vi "FL Fuzzy Controller (MIMO).vi"(8 "error in (no error)":errorcluster, 10 "input values":dbl[](array[numeric]), 11 "fuzzy system in":T1 {"user MF interpolating polynomials"."coa_x(y) coeff" format="%.4g"; "user MF interpolating polynomials"."Area(y) coeff" format="%.4g"; "user MF interpolating polynomials"."X(y) coeff" format="%.4g"; "user MF interpolating polynomials"."Y(x) coeff" format="%.4g"; "user MF interpolating polynomials"."Y" format="%.4g"; "user MF interpolating polynomials"."X" format="%.4g"; "defuzzification method" items=["Center of Area", "Modified Center of Area", "Center of Sums", "Center of Maximum", "Mean of Maximum"]; "rules"."consequents"."Var Index" min=0; "rules"."consequents"."Cond" items=["=", "!="]; "rules"."consequents"."MF Index" min=0; "rules"."antecedents"."Var Index" min=0; "rules"."antecedents"."Cond" items=["=", "!="]; "rules"."antecedents"."MF Index" min=0; "rules"."consequent implication" items=["Minimum", "Product"]; "rules"."antecedent connective" items=["AND (Minimum)", "AND (Product)", "OR (Maximum)", "OR (Probabilistic)"]; "output variables"."MFs"."shape" items=["Triangle", "Trapezoid", "Singleton", "Sigmoid", "Gaussian", "User-Defined"]; "input variables"."MFs"."shape" items=["Triangle", "Trapezoid", "Singleton", "Sigmoid", "Gaussian", "User-Defined"]}) -> (0 "error out":errorcluster, 1 "rule weights":dbl[](array[numeric]), 2 "output values":dbl[](array[numeric]), 3 "fuzzy system out":T1 {"user MF interpolating polynomials"."coa_x(y) coeff" format="%.4g"; "user MF interpolating polynomials"."Area(y) coeff" format="%.4g"; "user MF interpolating polynomials"."X(y) coeff" format="%.4g"; "user MF interpolating polynomials"."Y(x) coeff" format="%.4g"; "user MF interpolating polynomials"."Y" format="%.4g"; "user MF interpolating polynomials"."X" format="%.4g"; "defuzzification method" items=["Center of Area", "Modified Center of Area", "Center of Sums", "Center of Maximum", "Mean of Maximum"]; "rules"."consequents"."Var Index" min=0; "rules"."consequents"."Cond" items=["=", "!="]; "rules"."consequents"."MF Index" min=0; "rules"."antecedents"."Var Index" min=0; "rules"."antecedents"."Cond" items=["=", "!="]; "rules"."antecedents"."MF Index" min=0; "rules"."consequent implication" items=["Minimum", "Product"]; "rules"."antecedent connective" items=["AND (Minimum)", "AND (Product)", "OR (Maximum)", "OR (Probabilistic)"]; "output variables"."MFs"."shape" items=["Triangle", "Trapezoid", "Singleton", "Sigmoid", "Gaussian", "User-Defined"]; "input variables"."MFs"."shape" items=["Triangle", "Trapezoid", "Singleton", "Sigmoid", "Gaussian", "User-Defined"]}, 5 "rule-invoked values?":bool[](array[boolean]))   [LabVIEW 2017, in "NI_Fuzzy_Logic_API.lvlib"]
doc: "Implements a fuzzy logic controller for the fuzzy system you specify."
uses:
  <vilib>/addons/Fuzzy Logic/NI_Fuzzy_Logic_API.lvlib
  <vilib>/addons/Fuzzy Logic/TypeDefs/FL System.ctl
  <vilib>/addons/Fuzzy Logic/TypeDefs/FL Variable.ctl
  <vilib>/addons/Fuzzy Logic/TypeDefs/FL Membership Function.ctl
  <vilib>/addons/Fuzzy Logic/TypeDefs/FL Membership Function Shape.ctl
  <vilib>/addons/Fuzzy Logic/TypeDefs/FL Rule.ctl
  <vilib>/addons/Fuzzy Logic/TypeDefs/FL Antecedent.ctl
  <vilib>/addons/Fuzzy Logic/TypeDefs/FL Modifier.ctl
  <vilib>/addons/Fuzzy Logic/TypeDefs/FL Antecedent Connective.ctl
  <vilib>/addons/Fuzzy Logic/TypeDefs/FL Consequent.ctl
  <vilib>/addons/Fuzzy Logic/TypeDefs/FL Consequent Implication.ctl
  <vilib>/addons/Fuzzy Logic/TypeDefs/FL Defuzzification.ctl
  <vilib>/addons/Fuzzy Logic/TypeDefs/FL Interpolating polynomials.ctl
panel:
  # "IF"
  # "THEN"
  # "IF"
  # "THEN"
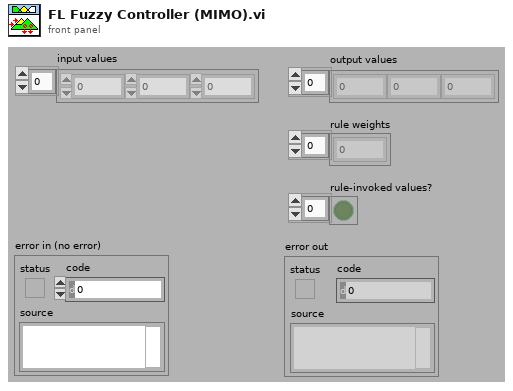
[diagram p1: front panel]
types:
  T1 = typedef "NI_Fuzzy_Logic_API.lvlib/FL System.ctl" = cluster{"input variables":T2[], "output variables":T2[], "rules":T5[], "defuzzification method":T11, "description":string, "user MF interpolating polynomials":T12[]}
  T2 = typedef "NI_Fuzzy_Logic_API.lvlib/FL Variable.ctl" = cluster{"name":string, "range":dbl[], "MFs":T3[]}
  T3 = typedef "NI_Fuzzy_Logic_API.lvlib/FL Membership Function.ctl" = cluster{"name":string, "shape":T4, "points":dbl[], "color":u32, "user-defined shape index":i32}
  T4 = typedef "NI_Fuzzy_Logic_API.lvlib/FL Membership Function Shape.ctl" = u16
  T5 = typedef "NI_Fuzzy_Logic_API.lvlib/FL Rule.ctl" = cluster{"antecedents":T6[], "antecedent connective":T8, "consequents":T9[], "consequent implication":T10, "degree of support":dbl}
  T6 = typedef "NI_Fuzzy_Logic_API.lvlib/FL Antecedent.ctl" = cluster{"Var Index":i32, "MF Index":i32, "Cond":T7}
  T7 = typedef "NI_Fuzzy_Logic_API.lvlib/FL Modifier.ctl" = u16
  T8 = typedef "NI_Fuzzy_Logic_API.lvlib/FL Antecedent Connective.ctl" = u16
  T9 = typedef "NI_Fuzzy_Logic_API.lvlib/FL Consequent.ctl" = cluster{"Var Index":i32, "MF Index":i32, "Cond":T7}
  T10 = typedef "NI_Fuzzy_Logic_API.lvlib/FL Consequent Implication.ctl" = u16
  T11 = typedef "NI_Fuzzy_Logic_API.lvlib/FL Defuzzification.ctl" = u16
  T12 = typedef "NI_Fuzzy_Logic_API.lvlib/FL Interpolating polynomials.ctl" = cluster{"X":dbl[], "Y":dbl[], "Y(x) coeff":dbl[][], "X(y) coeff":dbl[][], "Area(y) coeff":dbl[][], "coa_x(y) coeff":dbl[][]}
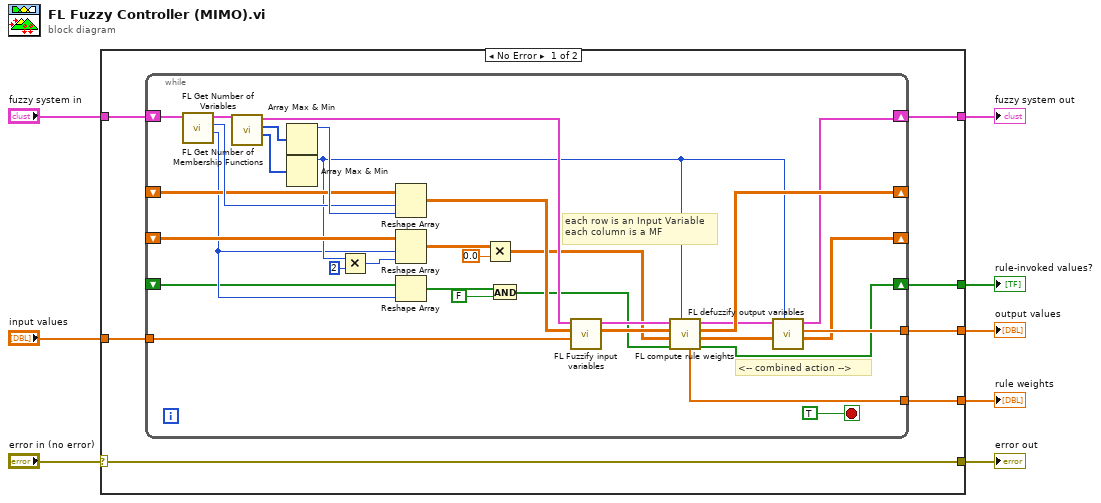
[diagram p0: block diagram]
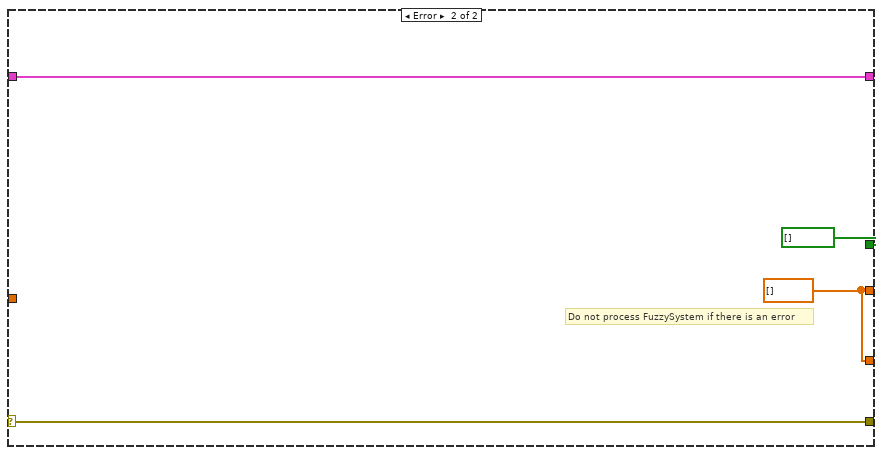
[diagram p2: hidden frame]
diagram:
  n1 = case shown="No Error" "error in (no error)" {
    selector: "error in (no error)" -> [w14 w51]
    tunnel: "fuzzy system in" -> [w12 w52]
    tunnel: [w15 w50] -> w7
    tunnel: [w14 w51] -> w6
    tunnel: [w10 w52] -> w4
    tunnel: "input values" -> [w13 _]
    tunnel: [w11 w50] -> w2
    tunnel: [w9 bool[] [] ("Array 2")] -> w1
    frame No Error {
      n2 = while {
        tunnel: [w44] -> w15
        tunnel: w13 -> [w47]
        shift-right: [w34] -> _
        shift-left: _ -> [w37]
        tunnel: [w43] -> w11
        shift-right: [w32] -> _
        shift-left: _ -> [w35]
        shift-right: [w28] -> w10
        shift-left: w12 -> [w38]
        shift-right: [w19] -> w9
        shift-left: _ -> [w20]
        stop <- TRUE stop-if-true
        # "<-- combined action -->"
        # "each row is an Input Variable\neach column is a MF"
        n3 = call <vilib>:"FL Get Number of Variables.vi"("fuzzy system in"=w38) -> ("number of output variables"=w21:i32, "number of input variables"=w40:i32, "fuzzy system out"=w39:T1)  [unwired: 1 in, 7 out]
        n4 = call <vilib>:"FL Get Number of Membership Functions.vi"("fuzzy system in"=w39) -> ("number of output membership functions"=w42:i32[], "number of input membership functions"=w41:i32[], "fuzzy system out"=w31:T1)  [unwired: 1 in, 7 out]
        n5 = Array Max & Min(array=w41) -> (max value=w48:i32)  [unwired: 3 out]
        n6 = Array Max & Min(array=w42) -> (max value=w24:i32)  [unwired: 3 out]
        n7 = Multiply(x=w24, y=2) -> (x*y=w25:i32)
        n8 = Reshape Array(w37, w40, w48) -> (w36:dbl[][])
        n9 = Reshape Array(w35, w21, w25) -> (w22:dbl[][])
        n10 = Reshape Array(w20, w21) -> (w17:bool[])
        n11 = Multiply(x=w22, y=0.0) -> (x*y=w27:dbl[][])
        n12 = And(x=w17, y=FALSE) -> (x .and. y?=w16:bool[])
        n13 = call <vilib>:"FL Fuzzify input variables.vi"("Input Variables"=w47, "input membership factors (u)"=w36, "fuzzy system in"=w31) -> ("membership factors (u)"=w46:dbl[][], "fuzzy system out"=w30:T1)  [unwired: 1 in, 6 out]
        n14 = call <vilib>:"FL compute rule weights.vi"("max num consequent membership functions"=w24, "rule-invoked array"=w16, "output membership factors (u)"=w27, "input membership factors (u)"=w46, "fuzzy system in"=w30) -> ("rule-invoked values?"=w19:bool[], "output membership factors (u)"=w33:dbl[][], "input membership factors (u)"=w34:dbl[][], "fuzzy system out"=w29:T1, "rule weights"=w43:dbl[])  [unwired: 2 out]
        n15 = call <vilib>:"FL defuzzify output variables.vi"("max num consequent membership fcns"=w24, "output membership factors (u)"=w33, "fuzzy system in"=w29) -> ("output membership factors (u)"=w32:dbl[][], "output variables"=w44:dbl[], "fuzzy system out"=w28:T1)  [unwired: 6 out]
      }
    }
    frame Error {
      w50 = dbl[] []
      # "Do not process FuzzySystem if there is an error"
    }
  }
  "fuzzy system out" <- w4
  "output values" <- w7
  "error out" <- w6
  "rule weights" <- w2
  "rule-invoked values?" <- w1
